vi "Swap Controllers.vi"(8 "error in (no error)":cluster{"状态":bool, "代码":i32, "源":string} caption="错误输入（无错误）", 10 "冷却器控制器":refnum<class "Cooler Controller.lvclass">, 11 "气冷系统应用程序输入":refnum<class "Air Cooler Application.lvclass">) -> (0 "error out":cluster{"状态":bool, "代码":i32, "源":string} caption="错误输出", 3 "气冷系统应用程序输出":refnum<class "Air Cooler Application.lvclass">)   [LabVIEW 2013, in "Air Cooler Application.lvlib" / "Air Cooler Application.lvclass"]
doc: "本VI负责更改当前正在运行的控制器操作者。输入的控制器将被启动，当前控制器将被停止。切换过程中冷却器将保持运行状态，不会被中断。"
uses:
  Air Cooler Application.lvclass
  Cooler Controller/Cooler Controller/Cooler Controller.lvclass
  <vilib>/ActorFramework/Actor/Actor.lvclass/Actor.ctl
  <vilib>/ActorFramework/Message Enqueuer/Message Enqueuer.lvclass/Message Enqueuer.ctl
  Air Cooler Application.lvclass/Air Cooler Application.ctl
  <vilib>/ActorFramework/Message Enqueuer/Message Enqueuer.lvclass
  <vilib>/ActorFramework/Message Enqueuer/Message Priority.ctl
  Cooler Controller/Write Cooler Enqueuer Msg/Write Cooler Enqueuer Msg.lvclass/Write Cooler Enqueuer Msg.ctl
  Cooler/Write Controller Enqueuer Msg/Write Controller Enqueuer Msg.lvclass/Write Controller Enqueuer Msg.ctl
  <vilib>/ActorFramework/Message Enqueuer/Init from Existing Queue.vi
  <vilib>/ActorFramework/Message Enqueuer/Enqueue.vi
  <vilib>/ActorFramework/Message Priority Queue/Priority Enqueue.vi
  Cooler Controller/Write Cooler Enqueuer Msg/Write Cooler Enqueuer Msg.lvclass
  Cooler/Write Controller Enqueuer Msg/Write Controller Enqueuer Msg.lvclass
  <vilib>/ActorFramework/Stop Msg/Stop Msg.lvclass
  <vilib>/ActorFramework/Actor/Actor.lvclass
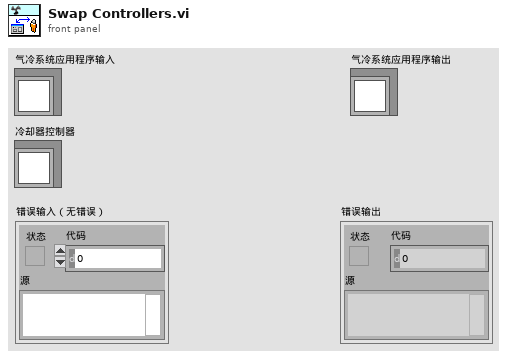
[diagram p1: front panel]
types:
  T1 = typedef "Actor Framework.lvlib/Message Enqueuer.lvclass/Message Priority.ctl" = enum16{"Low", "Normal", "High"}
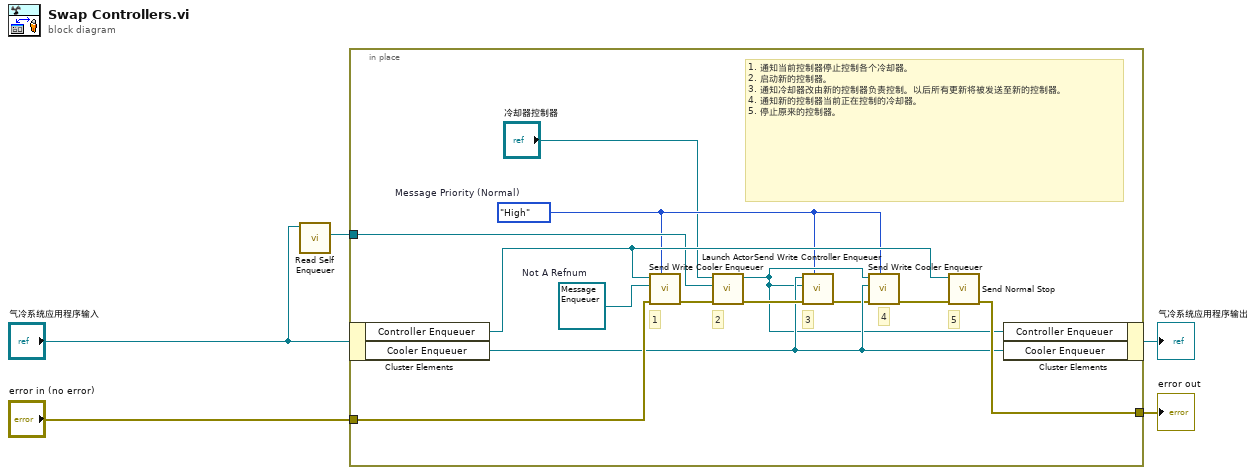
[diagram p0: block diagram]
diagram:
  n1 = call <vilib>:"Read Self Enqueuer.vi"("Actor"="气冷系统应用程序输入") -> ("Self Enqueuer"=w1:refnum<class "Message Enqueuer.lvclass">)  [unwired: 10 in]
  n2 = in-place {
    in-place-border: [w14] -> w4
    in-place-border: "error in (no error)" -> [w13]
    in-place-border: w1 -> [w12]
    w7 = Message_Priority."High"  # Message Priority (Normal)
    w17 = refnum<class "Message Enqueuer.lvclass"> refnum  # Not A Refnum
    # "4"
    # "1. 通知当前控制器停止控制各个冷却器。\n2. 启动新的控制器。\n3. 通知冷却器改由新的控制器负责控制。以后所有更新将被发送至新的控制器。\n4. 通知新的控制器当前正在控制的冷却器。\n5. 停止原来的控制器。"
    # "5"
    # "3"
    # "2"
    # "1"
    n3 = in-place-cluster #1("气冷系统应用程序输入") -> ("Controller Enqueuer"=w15:refnum<class "Message Enqueuer.lvclass">, "Cooler Enqueuer"=w11:refnum<class "Message Enqueuer.lvclass">)
    n4 = call "Send Write Cooler Enqueuer.vi"("消息优先级（标准）"=w7, "error in (no error)"=w13, "冷却器待入队列"=w17, "消息待入队列"=w15) -> ("error out"=w18:cluster{"状态":bool, "代码":i32, "源":string})  [unwired: 7 in]
    n5 = call <vilib>:"Launch Actor.vi"("error in (no error)"=w18, "Actor-to-Caller Enqueuer"=w12, "Actor"="冷却器控制器") -> ("error out"=w16:errorcluster, "Caller-To-Actor Enqueuer"=w10:refnum<class "Message Enqueuer.lvclass">)  [unwired: 7 in]
    n6 = call "Send Write Controller Enqueuer.vi"("消息优先级（标准）"=w7, "error in (no error)"=w16, "控制器待入队列"=w10, "消息待入队列"=w11) -> ("error out"=w9:cluster{"状态":bool, "代码":i32, "源":string})  [unwired: 7 in]
    n7 = call "Send Write Cooler Enqueuer.vi"("消息优先级（标准）"=w7, "error in (no error)"=w9, "冷却器待入队列"=w11, "消息待入队列"=w10) -> ("error out"=w8:cluster{"状态":bool, "代码":i32, "源":string})  [unwired: 7 in]
    n8 = call <vilib>:"Send Normal Stop.vi"("error in (no error)"=w8, "Message Enqueuer"=w15) -> ("error out"=w14:errorcluster)  [unwired: 9 in]
    n9 = in-place-cluster #1("Controller Enqueuer"=w10, "Cooler Enqueuer"=w11) -> (→"气冷系统应用程序输出":refnum<class "Air Cooler Application.lvclass">)
  }
  "error out" <- w4
